vi "Call Chain To Hash.vi"(1 "VI Call Chain":string[](array[string])) -> (0 "Key":string)   [LabVIEW 2009, in "Caraya.lvlib"]
uses:
  Caraya.lvlib
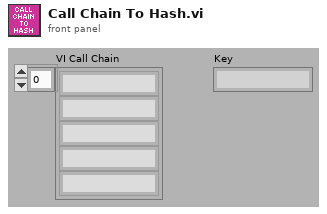
[diagram p1: front panel]
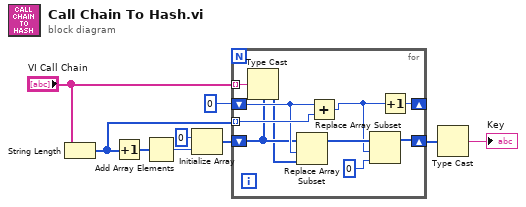
[diagram p0: block diagram]
diagram:
  n1 = String Length(string="VI Call Chain") -> (length=w1:i32[])
  n2 = Increment(x=w1) -> (x+1=w2:i32[])
  n3 = Add Array Elements(numeric array=w2) -> (sum=w3:i32)
  n4 = Initialize Array(u8 0 ("element"), w3) -> (w5:u8[])
  n5 = for {
    shift-right: [w12] -> w8
    shift-left: w5 -> [w16]
    tunnel: "VI Call Chain" -> [w17] mode=indexing
    shift-right: [w14] -> _
    shift-left: 0 -> [w18]
    tunnel: w1 -> [w19] mode=indexing
    n6 = Type Cast(type=w16, x=w17) -> (*(type *) &x=w15:u8[])
    n7 = Replace Array Subset(array=w16, new element=w15, index=w18) -> (w13:u8[])
    n8 = Add(x=w18, y=w19) -> (x+y=w11:i32)
    n9 = Replace Array Subset(array=w13, new element=u8 0 ("element"), index=w11) -> (w12:u8[])
    n10 = Increment(x=w11) -> (x+1=w14:i32)
  }
  n11 = Type Cast(x=w8) -> (*(type *) &x=→"Key":string)  [unwired: 1 in]
